vi "arrayAXRefs.vi"(0 "Array In":refnum<k7>[](array[refnum])) -> (1 "Number":dbl format="%0.2f", 2 "String":string, 3 "Cluster Out":cluster{"Numeric":dbl, "String":string} {"Numeric" format="%.2f"}, 4 "Array Out":refnum<k7>[](array[refnum]))   [LabVIEW 2011]
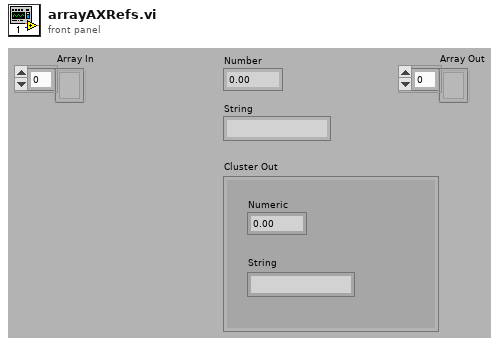
[diagram p1: front panel]
types:
  T1 = cluster{"GetValNumber":dbl, "GetValString":string}
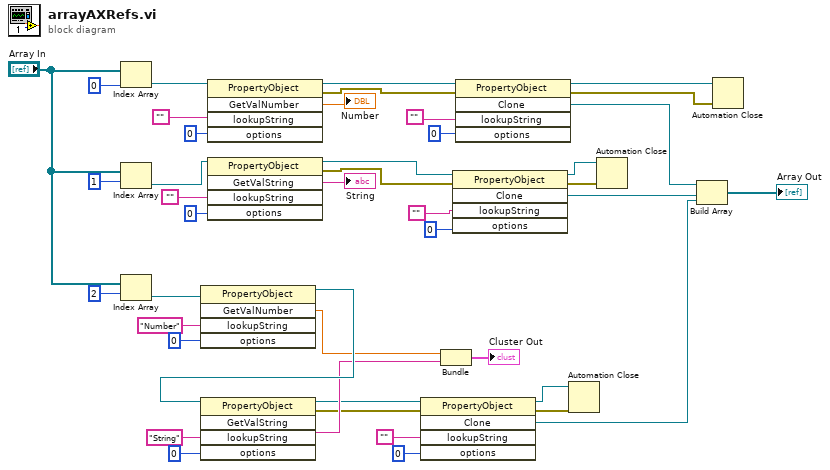
[diagram p0: block diagram]
diagram:
  n1 = Index Array(array="Array In", index=0) -> (element=w43:refnum<k7>)
  n2 = Index Array(array="Array In", index=1) -> (element=w12:refnum<k7>)
  n3 = Index Array(array="Array In", index=2) -> (element=w38:refnum<k7>)
  n4 = invoke class="PropertyObject" method="GetValNumber"(reference=w38, "lookupString"="Number", "options"=0) -> (reference out=w37:refnum<k7>, "GetValNumber"=w25:dbl)  [unwired: 2 in, 3 out]
  n5 = invoke class="PropertyObject" method="GetValString"(reference=w37, "lookupString"="String", "options"=0) -> (reference out=w7:refnum<k7>, error out=w6:errorcluster, "GetValString"=w24:string)  [unwired: 2 in, 2 out]
  n6 = invoke class="PropertyObject" method="GetValNumber"(reference=w43, "lookupString"="", "options"=0) -> (reference out=w23:refnum<k7>, error out=w21:errorcluster, "GetValNumber"=→"Number":dbl)  [unwired: 2 in, 2 out]
  n7 = invoke class="PropertyObject" method="GetValString"(reference=w12, "lookupString"="", "options"=0) -> (reference out=w13:refnum<k7>, error out=w11:errorcluster, "GetValString"=→"String":string)  [unwired: 2 in, 2 out]
  n8 = invoke class="PropertyObject" method="Clone"(reference=w7, error in=w6, "lookupString"="", "options"=0) -> (reference out=w5:refnum<k7>, error out=w4:errorcluster, "Clone"=w3:refnum<k7>)  [unwired: 1 in, 2 out]
  n9 = Bundle("GetValNumber"=w25, "GetValString"=w24) -> (→"Cluster Out":T1)  [unwired: 1 out]
  n10 = invoke class="PropertyObject" method="Clone"(reference=w13, error in=w11, "lookupString"="", "options"=0) -> (reference out=w15:refnum<k7>, error out=w14:errorcluster, "Clone"=w10:refnum<k7>)  [unwired: 1 in, 2 out]
  n11 = invoke class="PropertyObject" method="Clone"(reference=w23, error in=w21, "lookupString"="", "options"=0) -> (reference out=w22:refnum<k7>, error out=w20:errorcluster, "Clone"=w16:refnum<k7>)  [unwired: 1 in, 2 out]
  n12 = Automation Close(3:w4, 5:w5) -> ()  [unwired: 1 out]
  n13 = Automation Close(3:w14, 5:w15) -> ()  [unwired: 1 out]
  n14 = Build Array(w16, w10, w3) -> (→"Array Out":refnum<k7>[])
  n15 = Automation Close(3:w20, 5:w22) -> ()  [unwired: 1 out]
